vi "Mmap_Query.vi"(8 "error in (no error)":errorcluster, 11 "FAMM in":refnum<class "FAMM.lvclass">) -> (0 "error out":errorcluster, 3 "FAMM out":refnum<class "FAMM.lvclass">)   [LabVIEW 2020, in "Sgraph_lib_V1.lvlib" / "FAMM.lvclass"]
doc: "Andre Koelewijn, 3 april 2021\n\nThis VI will process a query as received from the Memory Map Visualizer.\nIt delivers an overvieuw of the buffer sizes and content"
uses:
  FAMM.lvclass
  Common/controls/MeMapInfo.ctl
  Common/controls/MMap_element.ctl
  Gserver/controls/Typedef_QueryType.ctl
  FAMM.lvclass/FAMM.ctl
  PAQ-memory.lvclass/PAQ-memory.ctl
  Gserver/Gserver.lvclass
  Builds/Sgraph_lib_V1.lvlib
  PAQ-memory.lvclass
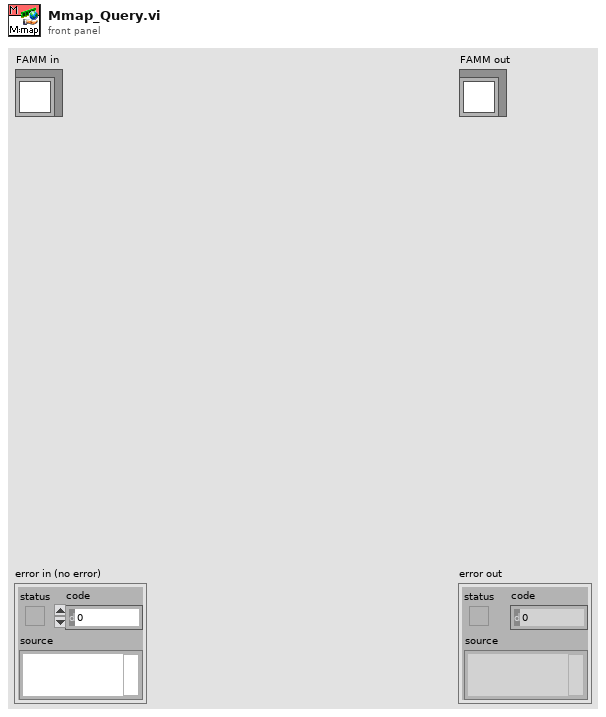
[diagram p1: front panel]
types:
  T1 = typedef "Sgraph_lib_V1.lvlib/Gserver.lvclass/Typedef_QueryType.ctl" = enum16{"Subscribe", "DataRequest", "RequestAllTags", "RequestIniPath", "FAMMstarted", "SetClientOptions", "GviewerUpdate", "OpenNewGraph", "CloseClient", "CloseAllClients", "Close Gserver", "OpenMemoryMap", "MeMapDataRequest", "MeMapDataResponse", "OpenDBeditor", "CheckDBeditorRunning", "StoppedDBeditor", "SaveDB_TAGpropRecord", "ConfirmDB_TAGpropSave"}
  T2 = typedef "Sgraph_lib_V1.lvlib/MeMapInfo.ctl" = cluster{"MemLayer":T3[]}
  T3 = typedef "Sgraph_lib_V1.lvlib/MMap_element.ctl" = cluster{"Name":string, "Length":i32, "Pointer":i32, "Tbegin":dbl, "Tend":dbl, "Tmin":dbl, "Tmax":dbl, "Tpnt-1":dbl, "Tpnt":dbl, "Tpnt+1":dbl, "Array":dbl[]}
  T4 = typedef "Sgraph_lib_V1.lvlib/FAMM.lvclass/FAMM-attributes.ctl" = cluster{"FAMM_PAQ_Layers":i32, "FAMM_PAQ_resolution":dbl, "PAQ_TAGs":string[], "WAQ_TAGs":string[], "EAQ_TAGs":string[], "All_TAGs":string[], "PAQtagProps":T5[], "WAQtagProps":T5[], "EAQtagProps":T5[], "DBAL_class":refnum<data-value>, "PAQ_memory":refnum<data-value>[], "PAQupdates":timestamp[], "FAMM_Size":cluster{"other":i32, "1day":i32, "1week":i32}, "DatabaseFileExtention":string, "DatabaseSaveRate":dbl, "Database_path":path, "DBAL-Queue":refnum<queue>, "OS_name":string}
  T5 = typedef "Sgraph_lib_V1.lvlib/typedef_com_TagProp.ctl" = cluster{"Description":string, "EngUnits":string, "RangeH":dbl, "RangeL":dbl, "Resolution":i32, "Obsolete":bool, "ChangeDate":timestamp, "ChangeSource":string, "ChangeReason":string, "TagFunc":u32}
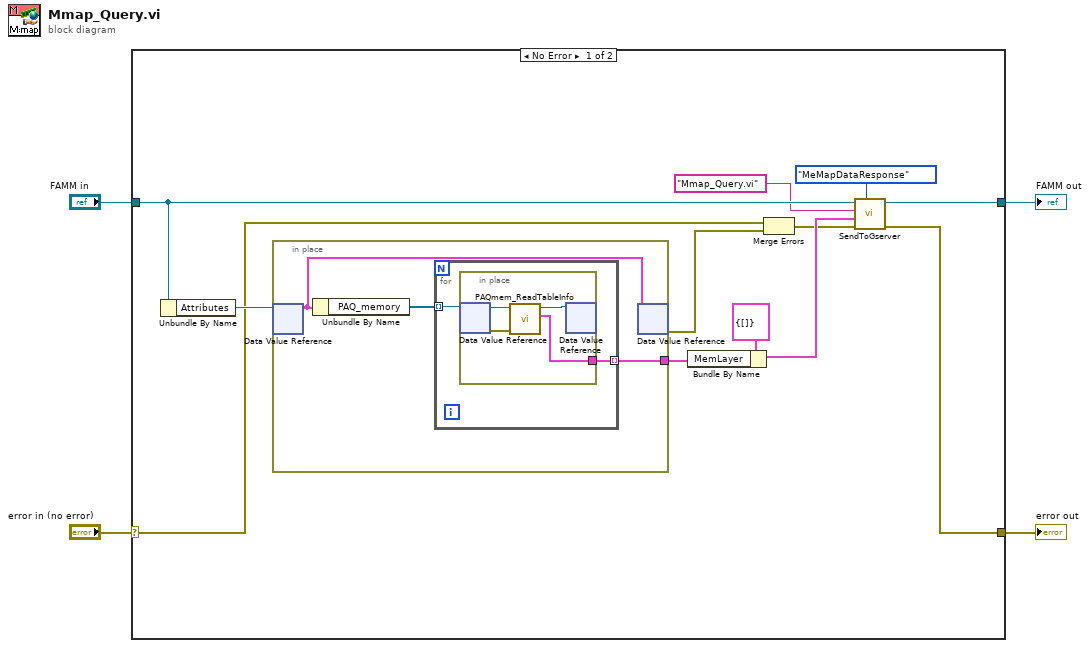
[diagram p0: block diagram]
diagram:
  n1 = case shown="No Error" "error in (no error)" {
    selector: "error in (no error)" -> [w9 w27]
    tunnel: [w6 w27] -> w3
    tunnel: [w7 w26] -> w1
    tunnel: "FAMM in" -> [w12 w26]
    frame No Error {
      n2 = Unbundle By Name(w12) -> ("Attributes"=w16:refnum<data-value>)
      n3 = in-place {
        in-place-border: [w19] -> w14
        n4 = in-place-dvr #1(w16) -> (w17:T4)  [unwired: 1 out]
        n5 = Unbundle By Name(w17) -> ("PAQ_memory"=w18:refnum<data-value>[])
        n6 = for {
          tunnel: w18 -> [w21] mode=indexing
          tunnel: [w20] -> w19 mode=indexing
          n7 = in-place {
            in-place-border: [w22] -> w20
            n8 = in-place-dvr #2(w21) -> (w25:refnum<class "PAQ-memory.lvclass">, w24:errorcluster)
            n9 = call "PAQmem_ReadTableInfo.vi"("error in (no error)"=w24, "PAQ-memory in"=w25) -> ("MemMap-element"=w22:T3, "PAQ-memory out"=w23:refnum<class "PAQ-memory.lvclass">)  [unwired: 7 in, 1 out]
            n10 = in-place-dvr #2(w23) -> ()  [unwired: 2 out]
          }
        }
        n11 = in-place-dvr #1(w17) -> (w10:errorcluster)  [unwired: 1 out]
      }
      n12 = Bundle By Name(cluster=T2 {"MemLayer"=[]} ("MemInfo"), "MemLayer"=w14) -> (w11:T2)
      n13 = Merge Errors(w9, w10) -> (w8:errorcluster)
      n14 = call "SendToGserver.vi"("Query_type"=Typedef_QueryType."MeMapDataResponse", "error in (no error)"=w8, "data"=w11, "Address"="Mmap_Query.vi", "FAMM in"=w12) -> ("error out"=w6:errorcluster, "FAMM out"=w7:refnum<class "FAMM.lvclass">)  [unwired: 5 in]
    }
    frame Error {
    }
  }
  "error out" <- w3
  "FAMM out" <- w1
